vi "Curved_Slot_Input.vi"(4 "error in (no error)":errorcluster, 5 "Measured origin x,y":dbl[](array[numeric])=[0.83, 0.79], 6 "Element In":T4, 7 "Outputmode":u16(ring) items=["Get Path", "Make Layout", "Create TRJs"]) -> (0 "error out":errorcluster, 1 "Init Cluster":T5, 2 "TRJs":T7, 3 "Elements Out":T6(array[cluster]))   [LabVIEW 2009]
panel:
  out "output cluster":T1
  in  "Tab Control":T2(tab)=enum."Output"
  in  "Length":dbl=11.0
  in  "interval between laser path":dbl=0.01
  in  "ablation rate":dbl=0.01
  in  "a0 radius":dbl=0.9
  in  "Remove distance":dbl=3.5
  in  "Height to groove":dbl=2.5
  in  "X distance from left edge":dbl=10.5
  in  "Slot geometry":cluster{bool, bool}
  in  "stop":bool
  in  "XY Line Arc Trajectory part 1":T3={"Velocity (units/s)"=3.0, "Acceleration (unts/s2)"=20.0, "Number of times of execution"=1} {"Acceleration (unts/s2)" format="%.6f"; "Velocity (units/s)" format="%.6f"; "Number of times of execution" format="%.6f"}
  in  "Type":i32=1
  # "This program always starts \nmachining from the center \nto the edge."
  # "Enter the distances of the horizontal and vertical lines from the sapphire edtes.\n\nFor gas slot power should be about 105mW with ablation rate 0.01, interval 0.01\n\nFor capillary power should be about 18-20mW with ablation rate 0.005, interval 0.008\nAlways a good idea to machine a few-mm capillary first to test ablation rate. Then\nadjust power linearly to make capillary round."
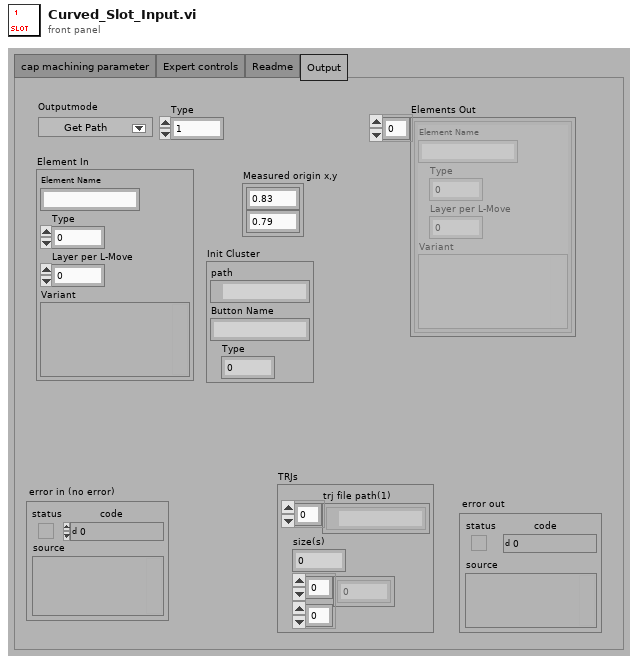
[diagram p1: front panel]
types:
  T1 = cluster{"element":dbl, "X distance from left edge":dbl, "Height to groove":dbl, "Remove distance":dbl, "a0 radius":dbl, "ablation rate":dbl, "interval between laser path":dbl, "Length ":dbl, "XY Line Arc Trajectory part 1":cluster{"Velocity (units/s)":dbl, "Acceleration (unts/s2)":dbl, "Number of times of execution":i32}, "Slot geometry":cluster{bool, bool}}
  T2 = enum32{"cap machining parameter", "Expert controls", "Readme", "Output"}
  T3 = cluster{"Velocity (units/s)":dbl, "Acceleration (unts/s2)":dbl, "Number of times of execution":i32}
  T4 = cluster{"Element Name":string, "Type":i32, "Layer per L-Move":i32, "Variant":variant}
  T5 = cluster{"path":path, "Button Name":string, "Type":i32}
  T6 = cluster{"Element Name":string, "Type":i32, "Layer per L-Move":i32, "Variant":variant}[]
  T7 = cluster{"trj file path(1)":path[], "size(s)":i32, dbl[][]}
  T8 = cluster{"Element Name":string, "Value":i32, "Layer per L-Move":i32, "Variant":variant}
  T9 = cluster{"Element Name":string, "Value":i32, "Layer per L-Move":i32, "Variant":variant}[]
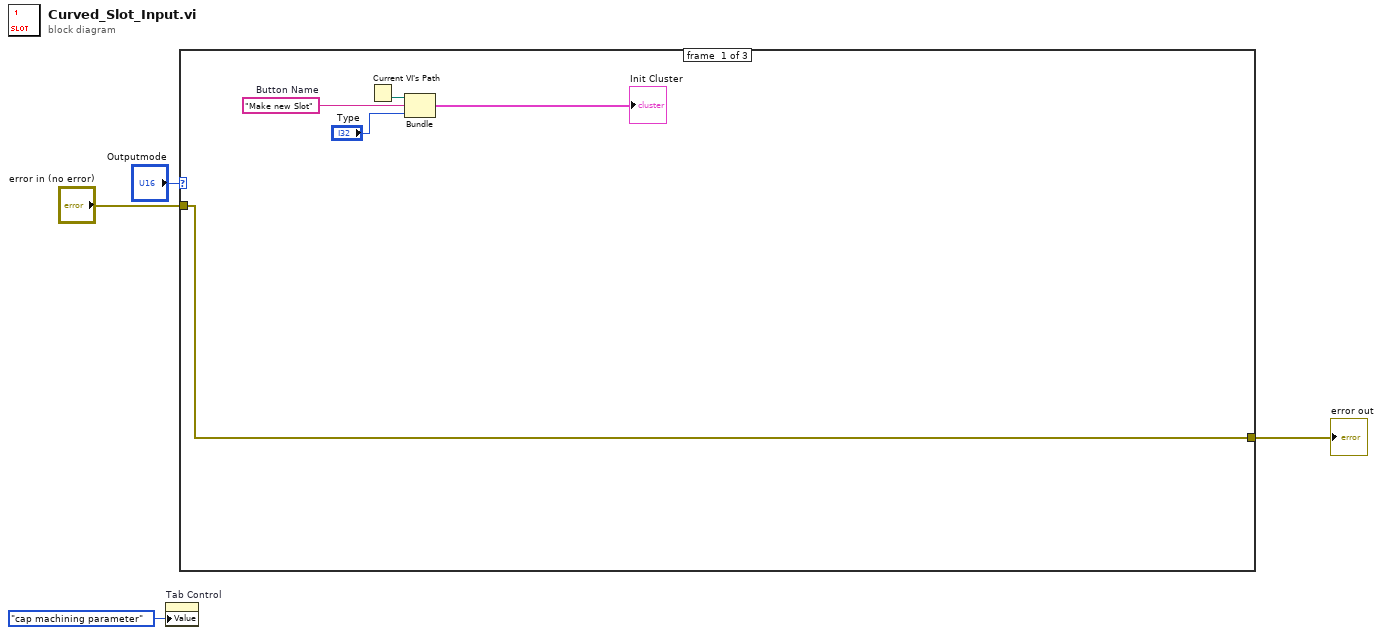
[diagram p0: block diagram]
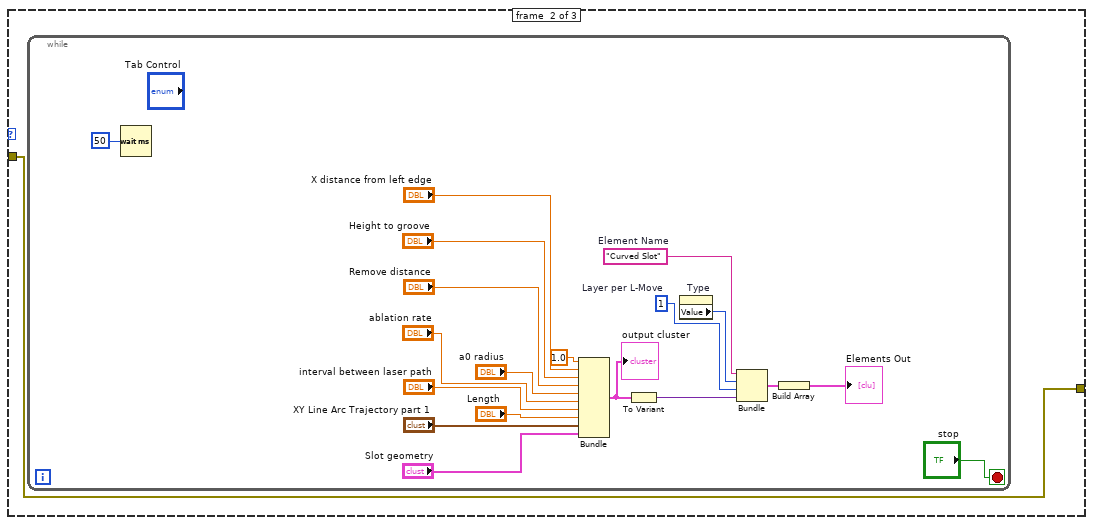
[diagram p2: hidden frame]
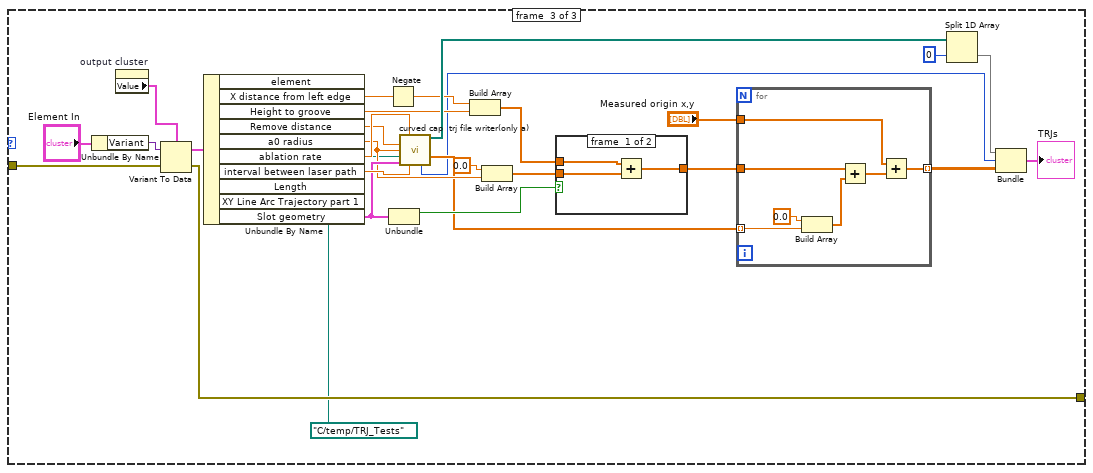
[diagram p3: hidden frame]
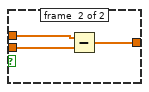
[diagram p4: hidden frame]
diagram:
  n1 = property on="Tab Control" class="TabCtl (strict)"("Value"=T2."cap machining parameter" ("Tab Control")) -> ()  [unwired: 2 in, 2 out]
  n2 = case shown="2" "Outputmode" {
    tunnel: "error in (no error)" -> [w5 w10 w53]
    tunnel: [w5 w10 w31] -> w1
    frame #0 {
      w7 = "Make new Slot"  # Button Name
      n3 = Current VI's Path() -> (path=w6:path)
      n4 = Bundle("path"=w6, "Button Name"=w7, "Type"="Type") -> (→"Init Cluster":T5)  [unwired: 1 in]
    }
    frame #1 {
      n5 = while {
        stop <- "stop" stop-if-true
        w16 = 1  # Layer per L-Move
        w13 = "Curved Slot"  # Element Name
        n6 = Wait (ms)(milliseconds to wait=u32 50) -> ()  [unwired: 1 out]
        n7 = Bundle("element"=1.0, "X distance from left edge"="X distance from left edge", "Height to groove"="Height to groove", "Remove distance"="Remove distance", "a0 radius"="a0 radius", "ablation rate"="ablation rate", "interval between laser path"="interval between laser path", "Length"="Length", "XY Line Arc Trajectory part 1"="XY Line Arc Trajectory part 1", "Slot geometry"="Slot geometry") -> (w12:T1)  [unwired: 1 in]
        "output cluster" <- w12
        n8 = To Variant(anything=w12) -> (Variant=w14:variant)
        n9 = property on="Type" class="DigNum (strict)"() -> ("Value"=w11:i32)  [unwired: 2 in, 2 out]
        n10 = Bundle("Element Name"=w13, "Value"=w11, "Layer per L-Move"=w16, "Variant"=w14) -> (w15:T8)  [unwired: 1 in]
        n11 = Build Array(w15) -> (→"Elements Out":T9)
      }
    }
    frame #2 {
      n12 = Unbundle By Name("Element In") -> ("Variant"=w56:variant)
      n13 = property on="output cluster" class="Clust (strict)"() -> ("Value"=w55:T1)  [unwired: 2 in, 2 out]
      n14 = Variant To Data(error in=w53, Variant=w56, type=w55) -> (error out=w31:errorcluster, data=w54:T1)
      n15 = Unbundle By Name(w54) -> ("X distance from left edge"=w41:dbl, "Height to groove"=w40:dbl, "Remove distance"=w51:dbl, "a0 radius"=w46:dbl, "ablation rate"=w52:dbl, "interval between laser path"=w50:dbl, "Slot geometry"=w47:cluster{bool, bool})  [unwired: 3 out]
      n16 = Negate(x=w41) -> (-x=w42:dbl)
      n17 = Unbundle(w47) -> (w39:bool)  [unwired: 1 out]
      n18 = call "curved cap  trj file writer(only a).vi"("ablation rate"=w52, "remove distance"=w51, "a0"=w46, "file (use dialog)"=path "C:/temp/TRJ_Tests", "Slot geometry"=w47, "interval between laser path"=w50) -> ("trj file path(1)"=w48:path[], "start point"=w37:dbl[], "size(s)"=w32:i32)  [unwired: 4 in, 3 out]
      n19 = Build Array(w42, w40) -> (w43:dbl[])
      n20 = Build Array(0.0 ("element"), w46) -> (w44:dbl[])
      n21 = case shown="False" w39 {
        tunnel: w44 -> [w66 w70]
        tunnel: w43 -> [w67 w69]
        tunnel: [w65 w68] -> w38
        frame #0 {
          n22 = Add(x=w67, y=w66) -> (x+y=w65:dbl[])
        }
        frame #1 {
          n23 = Subtract(x=w69, y=w70) -> (x-y=w68:dbl[])
        }
      }
      n24 = for {
        tunnel: w38 -> [w62]
        tunnel: w37 -> [w60] mode=indexing
        tunnel: "Measured origin x,y" -> [w59]
        tunnel: [w58] -> w34 mode=indexing
        n25 = Build Array(0.0 ("element"), w60) -> (w61:dbl[])
        n26 = Add(x=w62, y=w61) -> (x+y=w63:dbl[])
        n27 = Add(x=w59, y=w63) -> (x+y=w58:dbl[])
      }
      n28 = Split 1D Array(array=w48, index=0) -> (second subarray=w33:path[])  [unwired: 1 out]
      n29 = Bundle(w33, "size(s)"=w32, w34) -> (→"TRJs":cluster{path[], "size(s)":i32, dbl[][]})  [unwired: 1 in]
    }
  }
  "error out" <- w1
